vi "SRE Mask.vi"(7 "Mask":u8, 8 "error in (no error)":errorcluster, 10 "Node In":string, 11 "VISA resource name":refnum<visa-resource-name>) -> (0 "error out":errorcluster, 2 "Node Out":string, 3 "VISA resource name out":refnum<visa-resource-name>, 4 "Command String":string)   [LabVIEW 2013, in "Keithley 2600 Series.lvlib"]
doc: "Program the Service Request Enable Register. *SRE\n\n<b>Functions and Attributes Used</b>\nstatus.request_enable"
uses:
  Keithley 2600 Series.lvlib
panel:
  # "(c) 2008 Keithley Instruments, Inc.  ALL RIGHTS RESERVED."
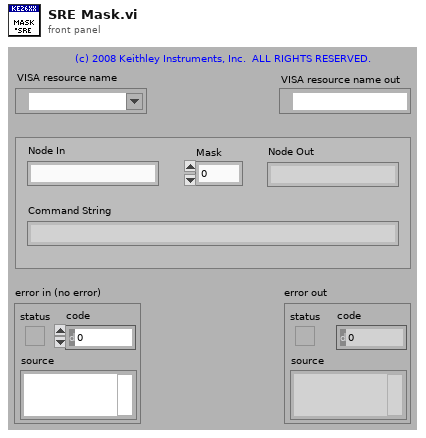
[diagram p1: front panel]
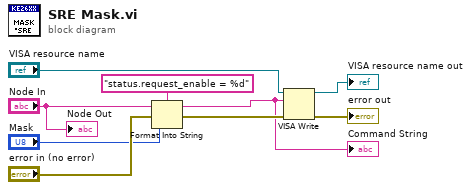
[diagram p0: block diagram]
diagram:
  n1 = Format Into String(format string="status.request_enable = %d", initial string="Node In", error in="error in (no error)", "Mask") -> (resulting string=w3:string, error out=w5:errorcluster)
  "Command String" <- w3
  n2 = VISA Write(VISA resource name="VISA resource name", write buffer=w3, error in (no error)=w5) -> (VISA resource name out=→"VISA resource name out":refnum<visa-resource-name>, error out=→"error out":errorcluster)  [unwired: 1 out]
  "Node Out" <- "Node In"
